vi "ChChangeSubV2.vi"(9 "data in":dbl[](array[numeric])) -> (1 "data out":dbl[](array[numeric]))   [LabVIEW 2020]
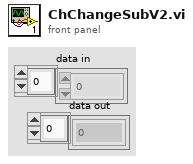
[diagram p1: front panel]
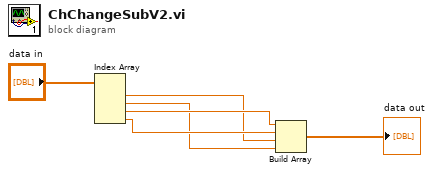
[diagram p0: block diagram]
diagram:
  n1 = Index Array(array="data in") -> (element #1=w3:dbl, element #2=w2:dbl, element #3=w5:dbl, element #4=w4:dbl)  [unwired: 4 in]
  n2 = Build Array(w5, w4, w3, w2) -> (→"data out":dbl[])
